vi "בדיקת מתח שחרור של סליל פיקוד ללא עומס 5.vi"(7 "resultUserPrompt":bool=TRUE, 8 "error":errorcluster, 10 "lines":tag="PXI1Slot8/port0/line1", 11 "Path for Log":path) -> (0 "error out":errorcluster, 1 "מצב ממסר פתוח/סגור":bool, 2 "מתח פתיחת הממסר":dbl format="%.4f", 3 "מתח מוצא מהספק":dbl format="%.4f")   [LabVIEW 2015]
uses:
  <vilib>/DAQmx/write.llb/DAQmx Write (Digital Bool 1Line 1Point).vi
  <vilib>/DAQmx/create/channels.llb/DAQmx Create Channel (DO-Digital Output).vi
  <vilib>/DAQmx/miscellaneous.llb/DAQmx Fill In Error Info.vi
panel:
  out "progress":dbl(slide) scale=0.0..11.0
  out "error IO DMM":errorcluster
  in  "Stop Button":bool
  # "Right-Click to\nexplain error"
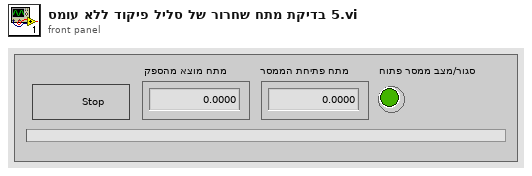
[diagram p1: front panel]
types:
  T1 = enum32{"Invalid", "Standard", "Closed", "Hidden", "Minimized", "Maximized"}
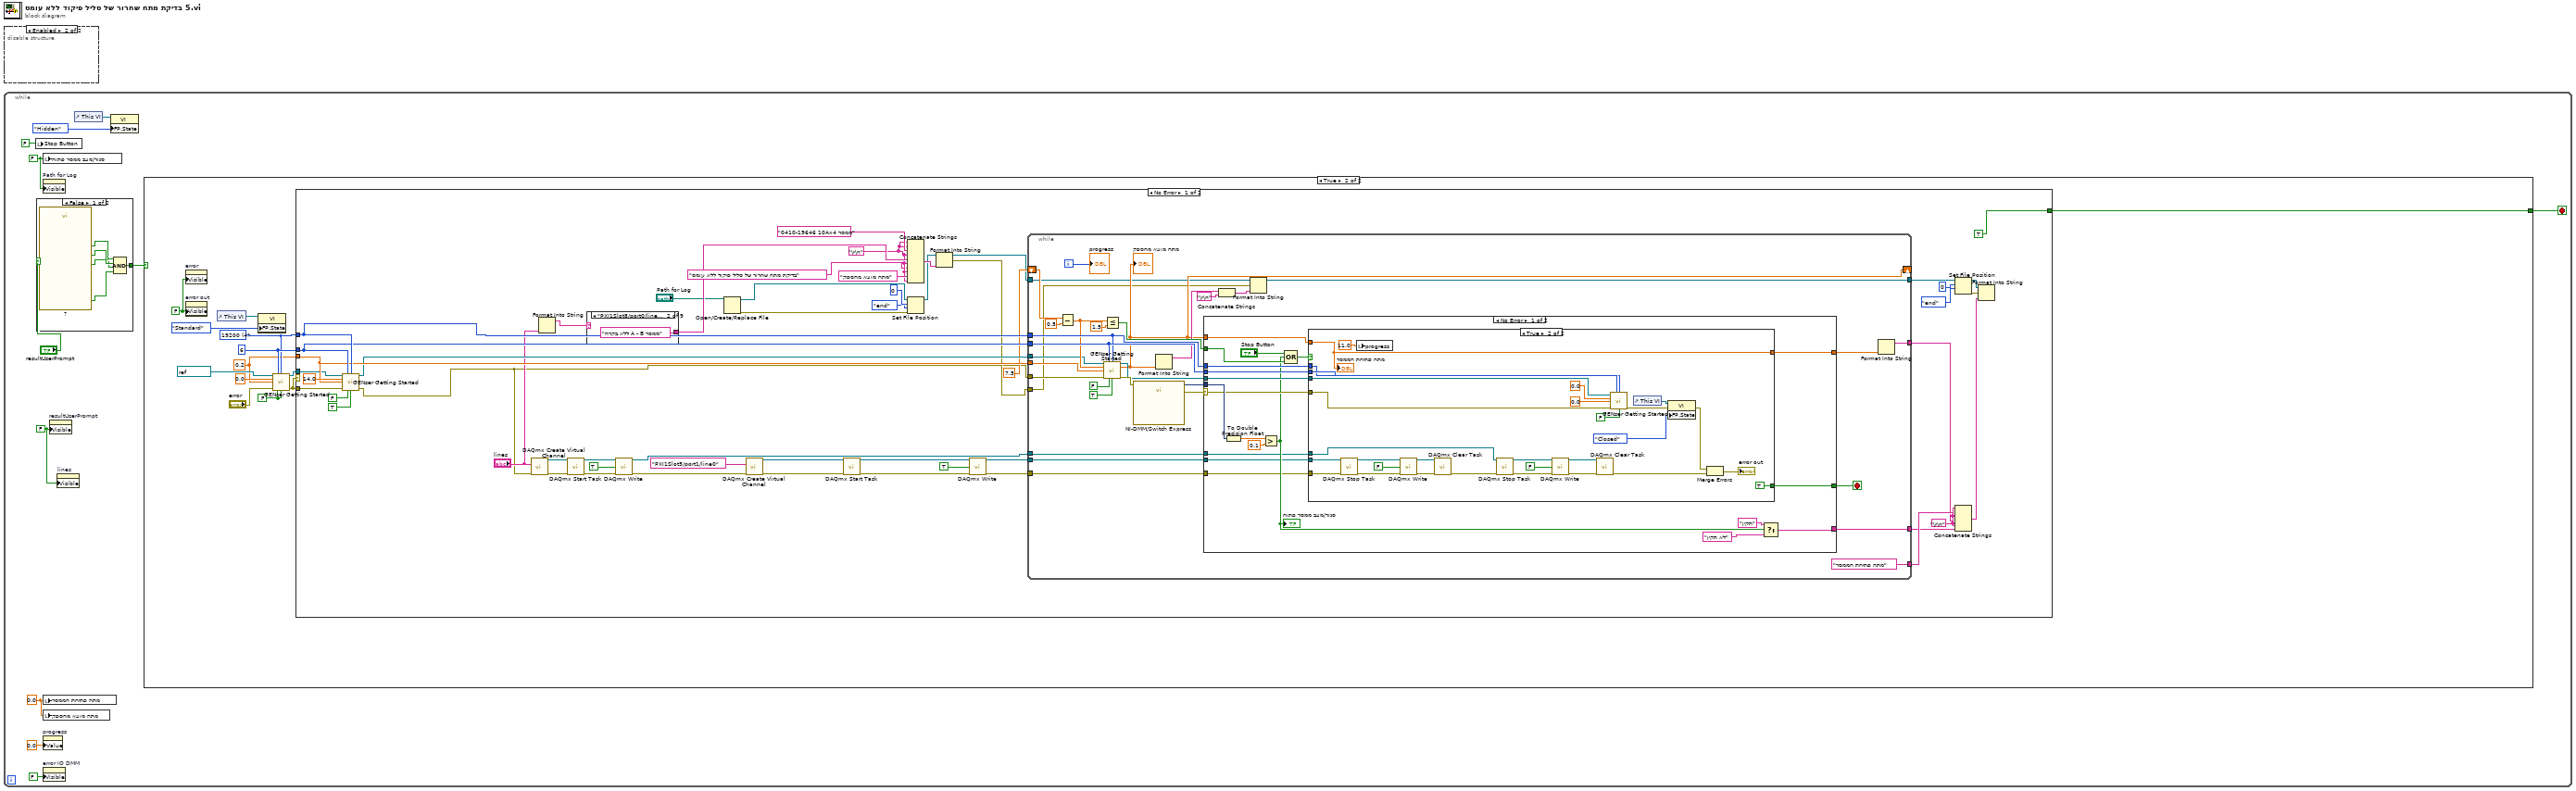
[diagram p0: block diagram]
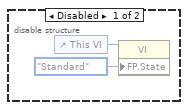
[diagram p2: hidden frame]
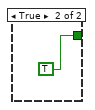
[diagram p3: hidden frame]
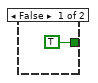
[diagram p4: hidden frame]
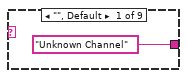
[diagram p5: hidden frame]
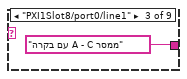
[diagram p6: hidden frame]
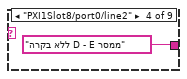
[diagram p7: hidden frame]
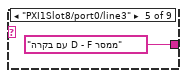
[diagram p8: hidden frame]
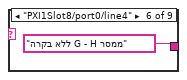
[diagram p9: hidden frame]
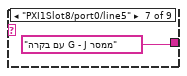
[diagram p10: hidden frame]
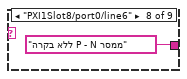
[diagram p11: hidden frame]
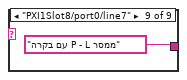
[diagram p12: hidden frame]
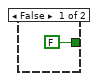
[diagram p13: hidden frame]
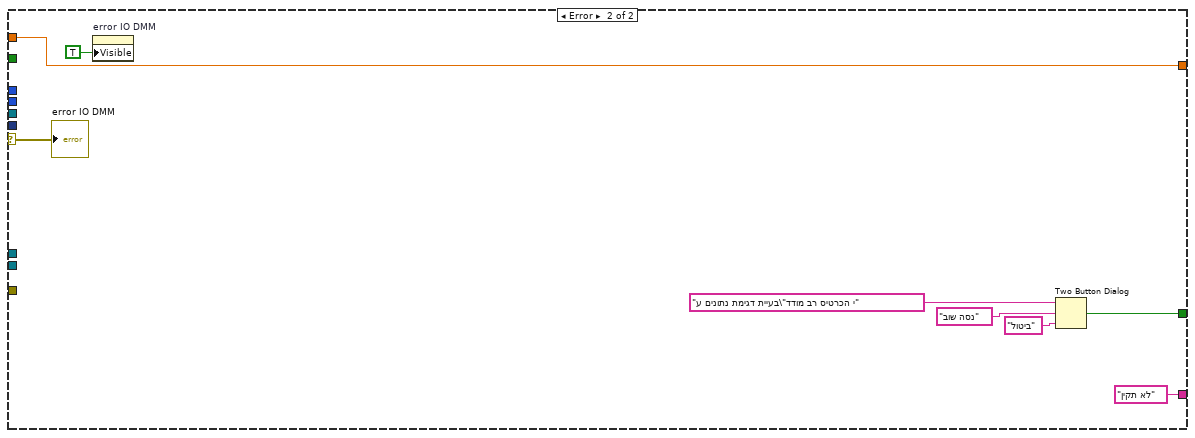
[diagram p14: hidden frame]
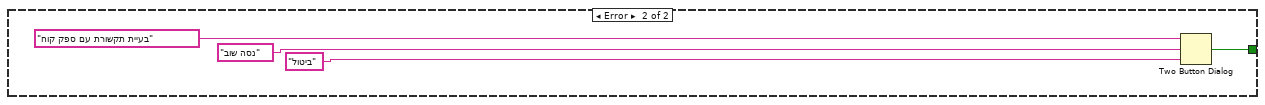
[diagram p15: hidden frame]
diagram:
  n1 = disable-structure shown="Enabled" {
    frame Disabled {
      n2 = control-ref of="This VI"() -> (w1:refnum<vi>)
      n3 = property class="VI"(reference=w1, "FP.State"=T1."Standard" ("Front Panel Window:State")) -> ()  [unwired: 1 in, 2 out]
    }
    frame Enabled {
    }
  }
  n4 = while {
    stop <- w3 stop-if-true
    w4 = FALSE ("Visible")
    w7 = FALSE ("מגע סגור")
    w10 = 0.0 ("signals out")
    n5 = local write "Stop Button"(FALSE ("Reset (T)")) -> ()
    n6 = case shown="False" "resultUserPrompt" {
      tunnel: [w18 TRUE] -> w5
      frame False {
        n7 = call "?"() -> ("הדקי הרב מודד"=w14:bool, "M מגע שלילי"=w15:bool, "K מגע חיובי"=w16:bool, "OK"=w17:bool)  [unwired: 15 in, 1 out]
        n8 = Compound Arithmetic op=AND(w17, w16, w15, w14) -> (w18:bool)
      }
      frame True {
      }
    }
    n9 = local write "מצב ממסר פתוח/סגור"(w7) -> ()
    n10 = property on="Path for Log" class="Path"("Visible"=w7) -> ()  [unwired: 2 in, 2 out]
    n11 = local write "מתח פתיחת הממסר"(w10) -> ()
    n12 = local write "מתח מוצא מהספק"(w10) -> ()
    n13 = property on="progress" class="Slide (strict)"("Value"=0.0 ("progress")) -> ()  [unwired: 2 in, 2 out]
    n14 = property on="error IO DMM" class="Clust (strict)"("Visible"=FALSE) -> ()  [unwired: 2 in, 2 out]
    n15 = property on="resultUserPrompt" class="Bool (strict)"("Visible"=w4) -> ()  [unwired: 2 in, 2 out]
    n16 = property on="lines" class="DAQmxName"("Visible"=w4) -> ()  [unwired: 2 in, 2 out]
    n17 = control-ref of="This VI"() -> (w9:refnum<vi>)
    n18 = property class="VI"(reference=w9, "FP.State"=T1."Hidden" ("Front Panel Window:State")) -> ()  [unwired: 1 in, 2 out]
    n19 = case shown="True" w5 {
      tunnel: [TRUE ("T button?") w25] -> w3
      frame False {
      }
      frame True {
        w23 = FALSE ("Visible")
        w24 = FALSE ("Output On (T)")
        w29 = u16 4 items=["1200", "2400", "4800", "9600", "19200"] ("BAUD")
        w30 = i16 6 ("GEN Addr")
        w26 = 0.2 ("Current Limit")
        n20 = property on="error" class="Clust (strict)"("Visible"=w23) -> ()  [unwired: 2 in, 2 out]
        n21 = property on="error out" class="Clust (strict)"("Visible"=w23) -> ()  [unwired: 2 in, 2 out]
        n22 = control-ref of="This VI"() -> (w21:refnum<vi>)
        n23 = property class="VI"(reference=w21, "FP.State"=T1."Standard" ("Front Panel Window:State")) -> ()  [unwired: 1 in, 2 out]
        n24 = call "GENser Getting Started.vi"("VISA"=refnum<visa-resource-name> "COM6", "GEN Addr"=w30, "BAUD"=w29, "Voltage Limit"=0.0, "Current Limit"=w26, "error"="error", "Reset (T)"=w24, "Output On (T)"=w24) -> ("VISA out"=w31:refnum<visa-resource-name>, "error out"=w32:errorcluster)  [unwired: 4 in, 2 out]
        n25 = case shown="No Error" w32 {
          tunnel: w32 -> [w83 _]
          tunnel: w31 -> [w79 _]
          tunnel: w30 -> [w81 _]
          tunnel: w29 -> [w82 _]
          tunnel: w26 -> [w80 _]
          tunnel: [TRUE w187] -> w25
          frame No Error {
            w40 = "\r\n"
            w75 = "\r\n"
            n26 = call "GENser Getting Started.vi"("VISA"=w79, "GEN Addr"=w81, "BAUD"=w82, "Voltage Limit"=14.0, "Current Limit"=w80, "error"=w83, "Reset (T)"=FALSE, "Output On (T)"=TRUE) -> ("VISA out"=w78:refnum<visa-resource-name>, "error out"=w34:errorcluster)  [unwired: 4 in, 2 out]
            n27 = call-poly <vilib>:"DAQmx Create Virtual Channel.vi"("lines"="lines", "error in"=w34) -> ("task out"=w57:refnum<k21>, "error out"=w56:errorcluster)  [unwired: 12 in]
            n28 = Format Into String("lines") -> (resulting string=w43:string)  [unwired: 3 in, 1 out]
            n29 = call <vilib>:"DAQmx Start Task.vi"("task/channels in"=w57, "error in"=w56) -> ("task out"=w54:refnum<k21>, "error out"=w55:errorcluster)  [unwired: 12 in]
            n30 = case shown="\"PXI1Slot8/port0/line0\"" w43 {
              tunnel: ["Unknown Channel" "ללא בקרה A - B ממסר" "עם בקרה A - C ממסר" "ללא בקרה D - E ממסר" "עם בקרה D - F ממסר" "ללא בקרה G - H ממסר" "עם בקרה G - J ממסר" "ללא בקרה P - N ממסר" "עם בקרה P - L ממסר"] -> w42
              frame "", Default {
              }
              frame "PXI1Slot8/port0/line0" {
              }
              frame "PXI1Slot8/port0/line1" {
              }
              frame "PXI1Slot8/port0/line2" {
              }
              frame "PXI1Slot8/port0/line3" {
              }
              frame "PXI1Slot8/port0/line4" {
              }
              frame "PXI1Slot8/port0/line5" {
              }
              frame "PXI1Slot8/port0/line6" {
              }
              frame "PXI1Slot8/port0/line7" {
              }
            }
            n31 = call-poly <vilib>:"DAQmx Write.vi"("task/channels in"=w54, "data"=TRUE, "error in"=w55) -> ("task out"=w51:refnum<k21>, "error out"=w52:errorcluster)  [unwired: 10 in, 1 out]
            n32 = Open/Create/Replace File(file path (use dialog)="Path for Log") -> (refnum out=w48:refnum<file>, error out=w47:errorcluster)  [unwired: 5 in, 1 out]
            n33 = call-poly <vilib>:"DAQmx Create Virtual Channel.vi"("lines"=tag "PXI1Slot5/port1/line0", "error in"=w52) -> ("task out"=w64:refnum<k21>, "error out"=w65:errorcluster)  [unwired: 12 in]
            n34 = call <vilib>:"DAQmx Start Task.vi"("task/channels in"=w64, "error in"=w65) -> ("task out"=w62:refnum<k21>, "error out"=w61:errorcluster)  [unwired: 12 in]
            n35 = Concatenate Strings(w40, w40, "0410-19646 10Ax4 ממסר", w40, w42, w40, "בדיקת מתח שחרור של סליל פיקוד ללא עומס", w40, "מתח מוצא מהספק", w40) -> (w46:string)
            n36 = Set File Position(offset (in bytes) (0)=i64 0, refnum=w48, from (0:start)=enum16{"start", "end", "current"}."end", error in=w47) -> (refnum out=w44:refnum<file>)  [unwired: 1 out]
            n37 = Format Into String(initial string=w44, w46) -> (resulting string=w35:refnum<file>, error out=w36:errorcluster)  [unwired: 2 in]
            n38 = call-poly <vilib>:"DAQmx Write.vi"("task/channels in"=w62, "data"=TRUE, "error in"=w61) -> ("task out"=w59:refnum<k21>, "error out"=w58:errorcluster)  [unwired: 10 in, 1 out]
            n39 = while {
              tunnel: w34 -> [w127]
              tunnel: w81 -> [w119]
              tunnel: w82 -> [w118]
              tunnel: w80 -> [w125]
              shift-right: [w101] -> _
              shift-left: 7.5 ("y") -> [w123]
              tunnel: w78 -> [w111]
              tunnel: [w106] -> w70
              tunnel: ["מתח פתיחת הממסר"] -> w69
              tunnel: [w104] -> w68
              tunnel: [w103] -> w67
              tunnel: w35 -> [w100]
              tunnel: w36 -> [w96]
              tunnel: w59 -> [w99]
              tunnel: w58 -> [w98]
              tunnel: w51 -> [w97]
              i -> [w112]
              stop <- w120 stop-if-true
              n40 = Subtract(x=w123, y=0.5) -> (x-y=w115:dbl)
              n41 = call "GENser Getting Started.vi"("VISA"=w111, "GEN Addr"=w119, "BAUD"=w118, "Voltage Limit"=w115, "Current Limit"=w125, "error"=w127, "Reset (T)"=FALSE, "Output On (T)"=TRUE) -> ("VISA out"=w117:refnum<visa-resource-name>, "Output Voltage"=w101:dbl, "error out"=w122:errorcluster)  [unwired: 4 in, 1 out]
              "מתח מוצא מהספק" <- w101
              n42 = Less Or Equal?(x=w115, y=1.5) -> (x <= y?=w114:bool)
              n43 = call "NI-DMM/Switch Express"("error in"=w122) -> ("signals out"=w121:dynamicdata, "error out"=w113:errorcluster)  [unwired: 16 in, 1 out]
              n44 = Format Into String(w101) -> (resulting string=w108:string)  [unwired: 3 in, 1 out]
              n45 = case shown="No Error" w113 {
                selector: w113 -> [w138 w186]
                tunnel: w121 -> [w147 _]
                tunnel: [w144 w182] -> w120
                tunnel: w119 -> [w143 _]
                tunnel: w118 -> [w142 _]
                tunnel: w117 -> [w141 _]
                tunnel: w114 -> [w140 _]
                tunnel: w101 -> [w139 w180]
                tunnel: [w132 w180] -> w107
                tunnel: [w131 "לא תקין"] -> w103
                tunnel: w99 -> [w130 _]
                tunnel: w98 -> [w129 _]
                tunnel: w97 -> [w128 _]
                frame No Error {
                  n46 = To Double Precision Float(number=w147) -> (double precision float=w137:dbl)
                  n47 = Greater?(x=w137, y=0.1) -> (0:w133:bool)
                  "מצב ממסר פתוח/סגור" <- w133
                  n48 = Compound Arithmetic op=OR("Stop Button", w133, w140) -> (w146:bool)
                  n49 = case shown="True" w146 {
                    tunnel: [FALSE TRUE] -> w144
                    tunnel: w143 -> [_ w177]
                    tunnel: w142 -> [_ w176]
                    tunnel: w141 -> [_ w175]
                    tunnel: w138 -> [_ w172]
                    tunnel: w139 -> [_ w166]
                    tunnel: [_ w166] -> w132
                    tunnel: w130 -> [_ w160]
                    tunnel: w129 -> [_ w159]
                    tunnel: w128 -> [_ w150]
                    frame False {
                    }
                    frame True {
                      n50 = call <vilib>:"DAQmx Stop Task.vi"("task/channels in"=w160, "error in"=w159) -> ("task out"=w165:refnum<k21>, "error out"=w164:errorcluster)  [unwired: 12 in]
                      n51 = local write "progress"(11.0 ("progress")) -> ()
                      n52 = call-poly <vilib>:"DAQmx Write.vi"("task/channels in"=w165, "data"=FALSE, "error in"=w164) -> ("task out"=w163:refnum<k21>, "error out"=w162:errorcluster)  [unwired: 10 in, 1 out]
                      n53 = call <vilib>:"DAQmx Clear Task.vi"("task in"=w163, "error in"=w162) -> ("error out"=w151:errorcluster)  [unwired: 13 in]
                      n54 = call <vilib>:"DAQmx Stop Task.vi"("task/channels in"=w150, "error in"=w151) -> ("task out"=w152:refnum<k21>, "error out"=w154:errorcluster)  [unwired: 12 in]
                      n55 = call-poly <vilib>:"DAQmx Write.vi"("task/channels in"=w152, "data"=FALSE, "error in"=w154) -> ("task out"=w155:refnum<k21>, "error out"=w156:errorcluster)  [unwired: 10 in, 1 out]
                      n56 = call <vilib>:"DAQmx Clear Task.vi"("task in"=w155, "error in"=w156) -> ("error out"=w149:errorcluster)  [unwired: 13 in]
                      n57 = call "GENser Getting Started.vi"("VISA"=w175, "GEN Addr"=w177, "BAUD"=w176, "Voltage Limit"=0.0, "Current Limit"=0.0, "error"=w172, "Output On (T)"=FALSE) -> ("error out"=w167:errorcluster)  [unwired: 5 in, 3 out]
                      n58 = control-ref of="This VI"() -> (w168:refnum<vi>)
                      n59 = property class="VI"(reference=w168, error in=w167, "FP.State"=T1."Closed" ("Front Panel Window:State")) -> (error out=w158:errorcluster)  [unwired: 1 out]
                      n60 = Merge Errors(w158, w149) -> (→"error out":errorcluster)
                      "מתח פתיחת הממסר" <- w166
                    }
                  }
                  n61 = Select(t="תקין", s=w133, f="לא תקין") -> (s? t:f=w131:string)
                }
                frame Error {
                  n62 = property on="error IO DMM" class="Clust (strict)"("Visible"=TRUE) -> ()  [unwired: 2 in, 2 out]
                  n63 = Two Button Dialog(message="בעיית דגימת נתונים ע\"י הכרטיס רב מודד", 1:"ביטול" ("F button name (\"Cancel\")"), 2:"נסה שוב" ("T button name (\"OK\")")) -> (T button?=w182:bool)
                  "error IO DMM" <- w186
                }
              }
              n64 = Concatenate Strings(w108, "\r\n") -> (w102:string)
              n65 = Format Into String(initial string=w100, error in=w96, w102) -> (resulting string=w106:refnum<file>)  [unwired: 1 in, 1 out]
              n66 = Format Into String(w107) -> (resulting string=w104:string)  [unwired: 3 in, 1 out]
              "progress" <- w112
            }
            n67 = Set File Position(offset (in bytes) (0)=i64 0, refnum=w70, from (0:start)=enum16{"start", "end", "current"}."end") -> (refnum out=w72:refnum<file>, error out=w71:errorcluster)  [unwired: 1 in]
            n68 = Concatenate Strings(w75, w69, w75, w68, w75, w67) -> (w66:string)
            n69 = Format Into String(initial string=w72, error in=w71, w66) -> ()  [unwired: 1 in, 2 out]
          }
          frame Error {
            n70 = Two Button Dialog(message="בעיית תקשורת עם ספק קוח", 1:"ביטול" ("F button name (\"Cancel\")"), 2:"נסה שוב" ("T button name (\"OK\")")) -> (T button?=w187:bool)
          }
        }
      }
    }
  }
